vi "H5Pget_dxpl_mpio.vi"(6 "error in (no error)":errorcluster, 9 "HDF5 Property Ref":T2) -> (0 "error out":errorcluster, 3 "HDF5 Ref out":T2, 8 "Xfer Mode":T1=1 items=["H5FD_MPIO_INDEPENDENT", "H5FD_MPIO_COLLECTIVE"])   [LabVIEW 2017]
doc: "Returns the data transfer mode."
uses:
  <vilib>/UPVI/lvhdf5/hdf5.dll
  <vilib>/UPVI/lvhdf5/library.llb/HDF5 Ref.ctl
  <vilib>/UPVI/lvhdf5/property.llb/H5FD_mpio_xfer_t.ctl
panel:
  # "LVHDF5 Toolkit\nCopyright (c) 2005-2013 by Jason D. Sommerville\nCopyright (c) 2014 by UPVI, LLC.\n\nThis use and distribution of this file is governed by the terms found in \nLICENSE.txt distributed with this toolkit and installed at\n <user.lib>\\_lvhdf5\\LICENSE.txt"
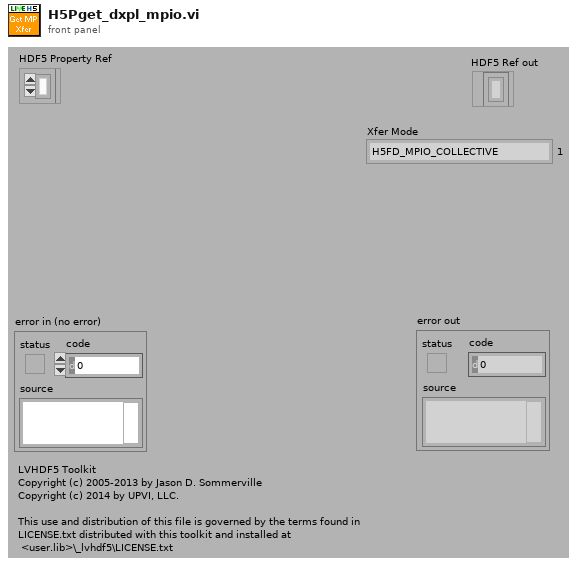
[diagram p1: front panel]
types:
  T1 = typedef "H5FD_mpio_xfer_t.ctl" = i32
  T2 = typedef "HDF5 Ref.ctl" = refnum<k1>
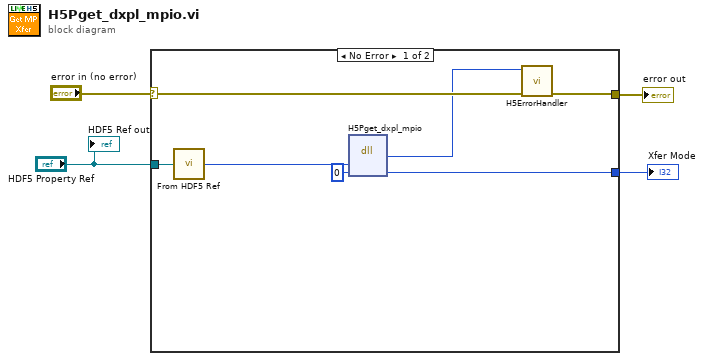
[diagram p0: block diagram]
diagram:
  n1 = case shown="No Error" "error in (no error)" {
    selector: "error in (no error)" -> [w11 w12]
    tunnel: [w10 w12] -> w3
    tunnel: "HDF5 Property Ref" -> [w8 _]
    tunnel: [w5 _] -> w1
    frame No Error {
      n2 = call <vilib>:"From HDF5 Ref.vi"("HDF5 Ref"=w8) -> ("I32"=w7:i32)
      n3 = dll-call lib="C:/Program Files/National Instruments/LabVIEW 2017/vi.lib/UPVI/lvhdf5/hdf5.dll" fn="H5Pget_dxpl_mpio"("plist_id"=w7, "xfer_mode"=0) -> (w9:u32, "xfer_mode"=w5:i32)  [unwired: 4 in, 2 out]
      n4 = call <vilib>:"H5ErrorHandler.vi"("error in (no error)"=w11, "herr_t"=w9) -> ("error out"=w10:errorcluster)  [unwired: 3 in, 4 out]
    }
    frame Error {
    }
  }
  "error out" <- w3
  "Xfer Mode" <- w1
  "HDF5 Ref out" <- "HDF5 Property Ref"
